vi "Forward Packet.vi"(10 "Response":T1, 11 "Session.Server in":refnum<class "Session.Server.lvclass">) -> (0 "error out":errorcluster)   [LabVIEW 2013, in "MQTT Server.lvlib" / "Session.Server.lvclass"]
uses:
  Session.Server.lvclass
  <vilib>/LabVIEW Open Source Project/MQTT Connection/MQTT_Base/Base Class/Response -- cluster.ctl
  <vilib>/LabVIEW Open Source Project/MQTT Control Packets/Control Packets/ControlPacket/ControlPacket.lvclass
  PacketCollection/PacketCollection.lvclass
  <vilib>/LabVIEW Open Source Project/MQTT Connection/MQTT_Base/Session/Session.lvclass
  <vilib>/LabVIEW Open Source Project/MQTT Connection/MQTT_Base/Base Class/MQTT_Base.lvclass
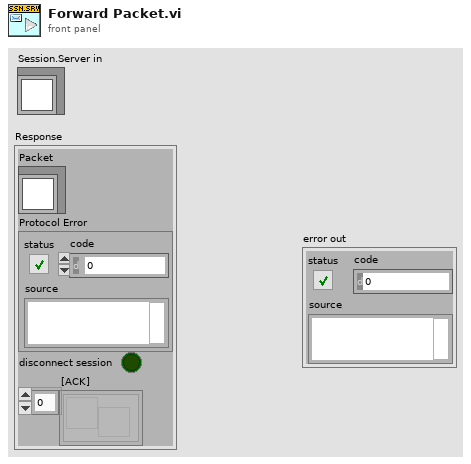
[diagram p1: front panel]
types:
  T1 = typedef "MQTT Base.lvlib/MQTT_Base.lvclass/Response -- cluster.ctl" = cluster{"Packet":refnum<class "ControlPacket.lvclass">, "Protocol Error":errorcluster, "disconnect session":bool, "[ACK]":refnum<notifier>[]}
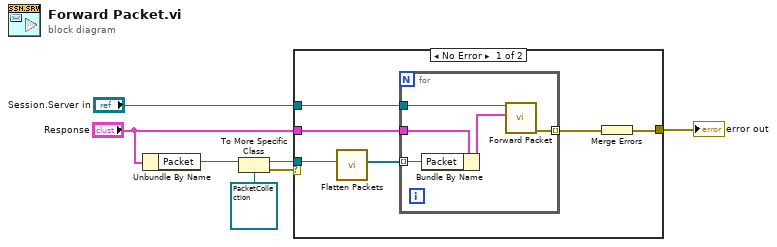
[diagram p0: block diagram]
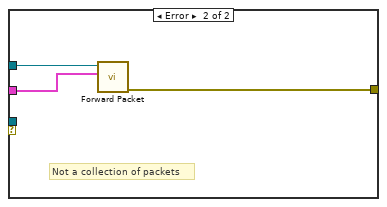
[diagram p2: hidden frame]
diagram:
  n1 = Unbundle By Name("Response") -> ("Packet"=w4:refnum<class "ControlPacket.lvclass">)
  n2 = To More Specific Class(target class=refnum<class "PacketCollection.lvclass"> refnum ("MQTT Server.lvlib:PacketCollection.lvclass"), reference=w4) -> (specific class reference=w1:refnum<class "PacketCollection.lvclass">, error out=w2:errorcluster)  [unwired: 1 in]
  n3 = case shown="No Error" w2 {
    tunnel: [w10 w21] -> w7
    tunnel: "Session.Server in" -> [w13 w20]
    tunnel: "Response" -> [w11 w19]
    tunnel: w1 -> [w9 _]
    frame No Error {
      n4 = call "Flatten Packets.vi"("Incoming Packet"=w9) -> ("Packets"=w8:refnum<class "ControlPacket.lvclass">[])  [unwired: 10 in]
      n5 = for {
        tunnel: w13 -> [w18]
        tunnel: [w17] -> w12 mode=indexing
        tunnel: w11 -> [w16]
        tunnel: w8 -> [w14] mode=indexing
        n6 = Bundle By Name(cluster=w16, "Packet"=w14) -> (w15:T1)
        n7 = call-parent "Forward Packet.vi"("Response"=w15, "Session in"=w18) -> ("error out"=w17:errorcluster)  [unwired: 9 in]
      }
      n8 = Merge Errors(w12) -> (w10:errorcluster)
    }
    frame Error {
      # "Not a collection of packets"
      n9 = call-parent "Forward Packet.vi"("Response"=w19, "Session in"=w20) -> ("error out"=w21:errorcluster)  [unwired: 9 in]
    }
  }
  "error out" <- w7
